vi "MALT132_005_TogleCommand_SlowInFiveSeconds.vi"() -> ()   [LabVIEW 2018]
uses:
  <instrlib>/Phi6/Common/Instrum/Phi6 Core/YAV-System.llb/YAV Info.ctl
  <instrlib>/Phi6/Common/Instrum/Phi6 Core/YAV-System.llb/YAV Card Total Info.ctl
  <instrlib>/Phi6/Common/Instrum/Phi6 Core/YAV-90132.llb/YAV90132 Mode Action.ctl
  <instrlib>/Phi6/Common/Instrum/Phi6 Core/YAV-90132.llb/YAV90132 Type Action.ctl
  <instrlib>/Phi6/Common/Instrum/Phi6 Core/CANNOU Global Variables.llb/CANNOU Global Variables.gbl.vi
panel:
  out "x-y":u32
  out "On &  Off Cycles":i32
  in  "stop":bool
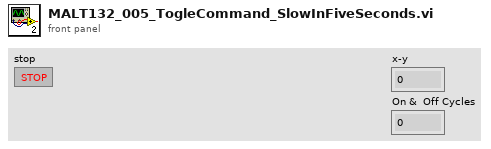
[diagram p1: front panel]
types:
  T1 = typedef "YAV Card Total Info.ctl" = cluster{"Index":u8, "Module":T2, "Version":u16, "Options":u8}
  T2 = typedef "YAV Info.ctl" = enum16{"-", "YAV90832", "YAV904X8", "YAV90132", "YAV91616", "YAV90PIN", "YAV90096", "YAV90HVT", "YAV90CLR", "YAV90128", "YAV90PNE", "YAVCANCON", "YAV91775", "YAV90XXX", "YAV90MMU", "H730050", "H710060", "H710061", "YAV90304", "MMI", "YAV90060", "YAV90MUX", "YAV90059", "YAV90070", "AK087", "Not Defined"}
  T3 = typedef "Module CAN.ctl" = enum16{"CAN0", "CAN1", "CAN2", "CAN3", "CAN4", "CAN5"}
  T4 = typedef "YAV90132 Type Action.ctl" = enum16{"None", "Set OFF", "Set ON", "TOGGLE", "BLINK", "PULSE ON", "PULSE OFF", "ASK", "Set OUT"}
  T5 = typedef "YAV90132 Mode Action.ctl" = enum16{"None", "One Relay", "Several Relays"}
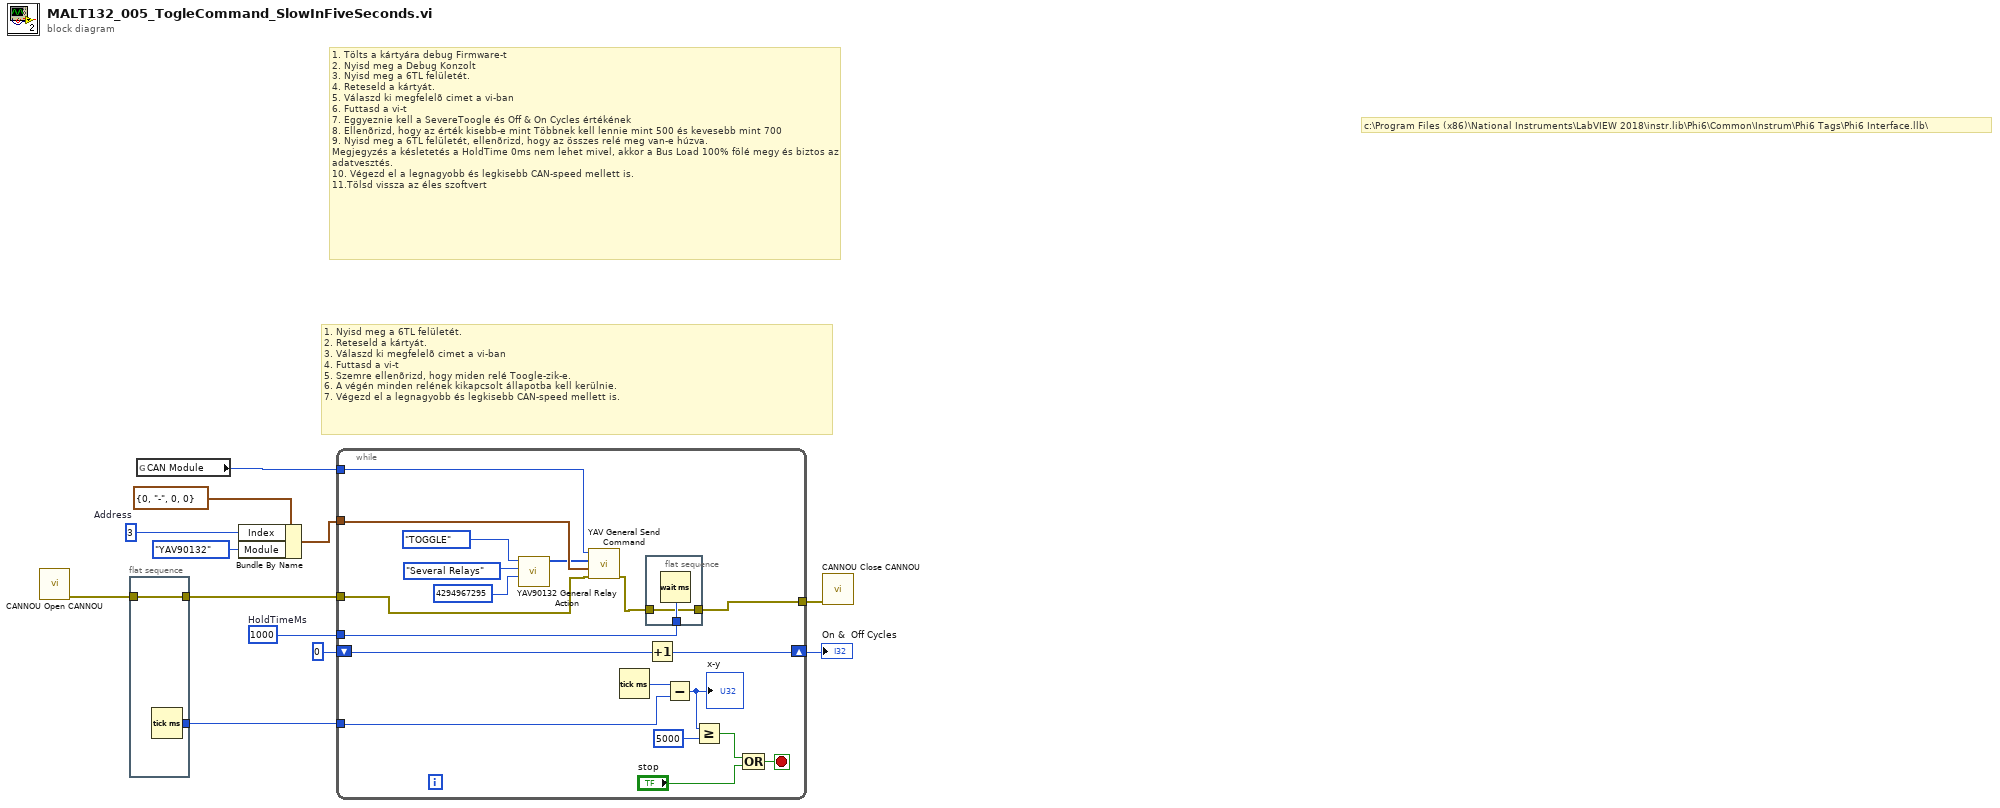
[diagram p0: block diagram]
diagram:
  w6 = u8 3  # Address
  w9 = 1000  # HoldTimeMs
  # "1. Tölts a kártyára debug Firmware-t\n2. Nyisd meg a Debug Konzolt\n3. Nyisd meg a 6TL felületét.\n4. Reteseld a kártyát.\n5. Válaszd ki megfelelõ cimet a vi-ban\n6. Futtasd a vi-t\n7. Eggyeznie kell a SevereToogle és Off & On Cycles értékének\n8. Ellenõrizd, hogy az érték kisebb-e mint Többnek kell lennie mint 500 és kevesebb mint 700\n9. Nyisd meg a 6TL felületét, ellenõrizd, hogy az összes relé meg van-e húzva.\nMegjegyzés a késletetés a HoldTime 0ms nem lehet mivel, akkor a Bus Load 100% fölé megy és biztos az adatvesztés.\n10. Végezd el a legnagyobb és legkisebb CAN-speed mellett is.\n11.Tölsd vissza az éles szoftvert"
  # "1. Nyisd meg a 6TL felületét.\n2. Reteseld a kártyát.\n3. Válaszd ki megfelelõ cimet a vi-ban\n4. Futtasd a vi-t\n5. Szemre ellenõrizd, hogy miden relé Toogle-zik-e.\n6. A végén minden relének kikapcsolt állapotba kell kerülnie.\n7. Végezd el a legnagyobb és legkisebb CAN-speed mellett is."
  # "c:\\Program Files (x86)\\National Instruments\\LabVIEW 2018\\instr.lib\\Phi6\\Common\\Instrum\\Phi6 Tags\\Phi6 Interface.llb\\"
  n1 = call <instrlib>:"CANNOU Open CANNOU.vi"() -> ("error out"=w1:errorcluster)  [unwired: 6 in, 1 out]
  n2 = flat-sequence {
    tunnel: [w14] -> w10
    tunnel: [w13] -> w2
    tunnel: w1 -> [w13]
    frame #0 {
      n3 = Tick Count (ms)() -> (millisecond timer value=w14:u32)
    }
  }
  n4 = global read "CANNOU Global Variables.gbl.vi" "CAN Module"() -> (w3:T3)
  n5 = Bundle By Name(cluster=T1 {"Index"=0, "Module"=enum."-", "Version"=0, "Options"=0} ("Info In"), "Index"=w6, "Module"=YAV_Info."YAV90132") -> (w5:T1)
  n6 = while {
    shift-right: [w32] -> w11
    shift-left: 0 -> [w33]
    tunnel: w10 -> [w30]
    tunnel: w9 -> [w24]
    tunnel: w5 -> [w23]
    tunnel: w2 -> [w22]
    tunnel: [w15] -> w4
    tunnel: w3 -> [w17]
    stop <- w25 stop-if-true
    n7 = call <instrlib>:"YAV90132 General Relay Action.vi"("Relay/Relays"=u32 4294967295, "Mode Action"=YAV90132_Mode_Action."Several Relays", "Type Action"=YAV90132_Type_Action."TOGGLE") -> ("Data"=w18:u8[])  [unwired: 8 in]
    n8 = call <instrlib>:"YAV General Send Command.vi"("error in"=w22, "Info In"=w23, "Data"=w18, "CAN Module"=w17) -> ("error out"=w16:errorcluster)  [unwired: 2 in, 1 out]
    n9 = Tick Count (ms)() -> (millisecond timer value=w31:u32)
    n10 = flat-sequence {
      tunnel: w24 -> [w35]
      tunnel: [w34] -> w15
      tunnel: w16 -> [w34]
      frame #0 {
        n11 = Wait (ms)(milliseconds to wait=w35) -> ()  [unwired: 1 out]
      }
    }
    n12 = Increment(x=w33) -> (x+1=w32:i32)
    n13 = Subtract(x=w31, y=w30) -> (x-y=w29:u32)
    "x-y" <- w29
    n14 = Greater Or Equal?(x=w29, y=u32 5000) -> (x >= y?=w27:bool)
    n15 = Compound Arithmetic op=OR(w27, "stop") -> (w25:bool)
  }
  "On &  Off Cycles" <- w11
  n16 = call <instrlib>:"CANNOU Close CANNOU.vi"("error in"=w4) -> ()  [unwired: 6 in, 1 out]
